vi "Speed Test.vi"() -> ()   [LabVIEW 2021]
panel:
  out "Mes Pos (mm)":dbl[](array[slide]) scale=-1200.0..-500.0
  out "RPM":dbl[](array[knob]) scale=-200.0..200.0
  in  "stop":bool
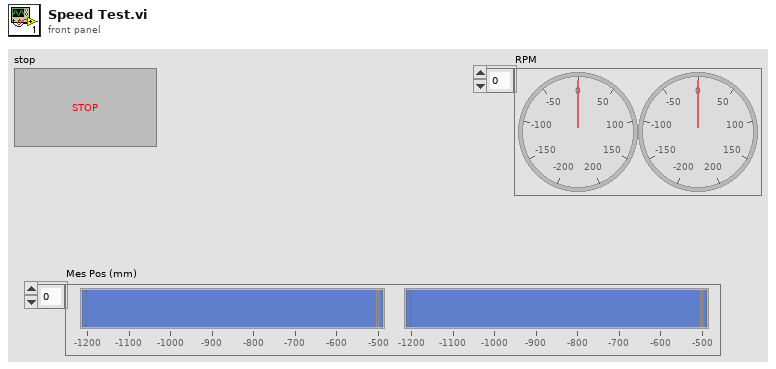
[diagram p1: front panel]
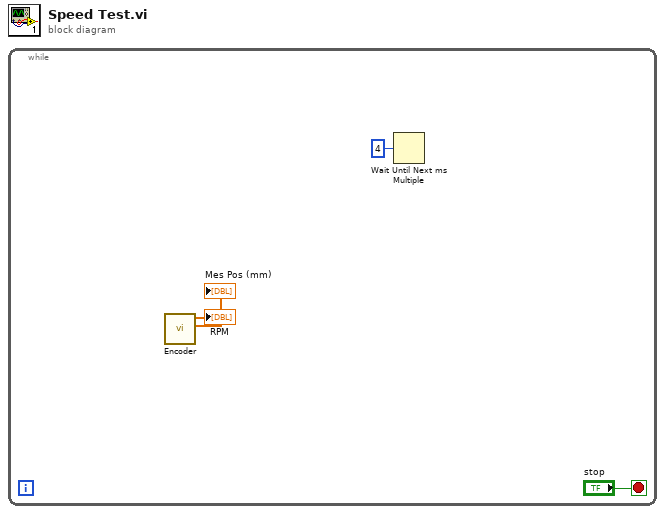
[diagram p0: block diagram]
diagram:
  n1 = while {
    stop <- "stop" stop-if-true
    n2 = call "Encoder.vi"() -> ("Mes Pos (mm)"=→"Mes Pos (mm)":dbl[], "RPM"=→"RPM":dbl[])  [unwired: 10 in]
    n3 = Wait Until Next ms Multiple(millisecond multiple=u32 4) -> ()  [unwired: 1 out]
  }
